vi "Review Intermediate Results.vi"(0 "Intermediate Results":string, 5 "Request Message":string, 9 "Request Header":string, 11 "error in (no error)":errorcluster) -> (4 "Response":string, 15 "error out":errorcluster)   [LabVIEW 2023, in "RFCalAndFixtureCharact.Common.lvlib"]
uses:
  RFCalAndFixtureCharact.Common.lvlib
  C:/srd-semi-rfcal-software/AuxTools/STSRFFixtureCharactUtility/Source/Code Modules/Dependencies/NationalInstruments.RFCalibration.ExecutionEngine.dll
  Dependencies/NationalInstruments.RFCalibration.ExecutionEngine.dll
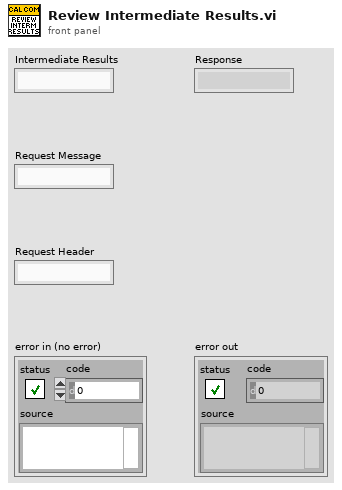
[diagram p1: front panel]
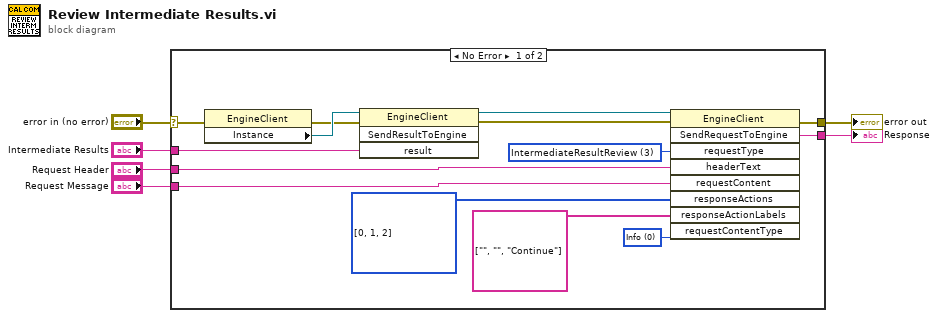
[diagram p0: block diagram]
diagram:
  n1 = case shown="No Error" "error in (no error)" {
    selector: "error in (no error)" -> [w18 w21]
    tunnel: [w20 w21] -> w6
    tunnel: [w19 _] -> w5
    tunnel: "Request Header" -> [w17 _]
    tunnel: "Request Message" -> [w16 _]
    tunnel: "Intermediate Results" -> [w12 _]
    frame No Error {
      w7 = 0 items=["Info", "Warning", "Error", "Action"] ("requestContentType")
      w9 = i32[] [0, 1, 2] items=["Abort", "Retry", "Continue", "Skip"] ("responseActions")
      w10 = 3 items=["Command", "ResultConfirmation", "CheckListenerStatus", "IntermediateResultReview"] ("Request Type")
      n2 = property class="EngineClient"(error in=w18) -> (error out=w11:errorcluster, "Instance"=w15:refnum<k24>)  [unwired: 1 in, 1 out]
      n3 = invoke class="EngineClient" method="SendResultToEngine"(reference=w15, error in=w11, "result"=w12) -> (reference out=w14:refnum<k24>, error out=w13:errorcluster)  [unwired: 1 in, 2 out]
      n4 = invoke class="EngineClient" method="SendRequestToEngine"(reference=w14, error in=w13, "requestType"=w10, "headerText"=w17, "requestContent"=w16, "responseActions"=w9, "responseActionLabels"=string[] ["", "", "Continue"], "requestContentType"=w7) -> (error out=w20:errorcluster, "SendRequestToEngine"=w19:string)  [unwired: 1 in, 7 out]
    }
    frame Error {
    }
  }
  "error out" <- w6
  "Response" <- w5
